vi "Timer.vi"(8 "Info:":string, 11 "SetTime":dbl) -> ()   [LabVIEW 2012]
panel:
  in  "停止":bool
  out "Last Info":string
  out "Timer-":i64
  out "Time+":i64 caption="Timer"
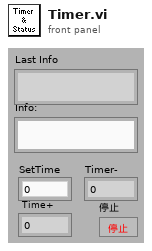
[diagram p1: front panel]
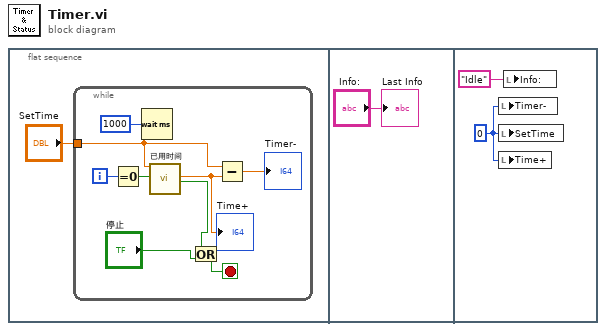
[diagram p0: block diagram]
diagram:
  n1 = flat-sequence {
    frame #0 {
      n2 = while {
        tunnel: "SetTime" -> [w9]
        i -> [w6]
        stop <- w2 stop-if-true
        n3 = Equal To 0?(x=w6) -> (x = 0?=w5:bool)
        n4 = Wait (ms)(milliseconds to wait=u32 1000 ("等待时间（毫秒）")) -> ()  [unwired: 1 out]
        n5 = call "已用时间"("Time Target (s)"=w9, "Reset"=w5) -> ("Elapsed Time (s)"=w8:dbl, "Time has Elapsed"=w3:bool)  [unwired: 10 in, 6 out]
        "Time+" <- w8
        n6 = Or(x=w3, y="停止") -> (x .or. y?=w2:bool)
        n7 = Subtract(x=w9, y=w8) -> (x-y=→"Timer-":dbl)
      }
    }
    frame #1 {
      "Last Info" <- "Info:"
    }
    frame #2 {
      w13 = i16 0 ("Timer-")
      n8 = local write "Timer-"(w13) -> ()
      n9 = local write "SetTime"(w13) -> ()
      n10 = local write "Time+"(w13) -> ()
      n11 = local write "Info:"("Idle" ("Info:")) -> ()
    }
  }
